vi "PullZeros.vi"(4 "input":dbl[](array[numeric]) format="%.2f") -> (0 "output":dbl[](array[numeric]) format="%.2f", 1 "non zero points":i32, 2 "pre-zeros":i32)   [LabVIEW 2022 SP3]
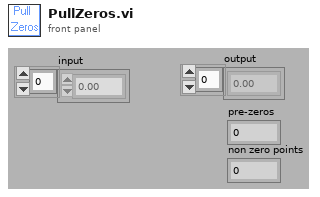
[diagram p1: front panel]
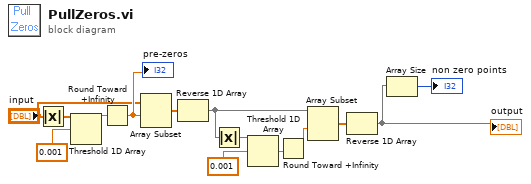
[diagram p0: block diagram]
diagram:
  n1 = Absolute Value(x="input") -> (abs(x)=w3:dbl[])
  n2 = Threshold 1D Array(2:0.001, 3:w3) -> (0:w10:dbl)  [unwired: 1 out]
  n3 = Round Toward +Infinity(x=w10) -> (ceil(x): smallest int >= x=w14:dbl)
  "pre-zeros" <- w14
  n4 = Array Subset(array="input", index=w14) -> (w4:dbl[])  [unwired: 1 in]
  n5 = Reverse 1D Array(array=w4) -> (reversed array=w7:dbl[])
  n6 = Absolute Value(x=w7) -> (abs(x)=w6:dbl[])
  n7 = Threshold 1D Array(2:0.001, 3:w6) -> (0:w9:dbl)  [unwired: 1 out]
  n8 = Round Toward +Infinity(x=w9) -> (ceil(x): smallest int >= x=w12:dbl)
  n9 = Array Subset(array=w7, index=w12) -> (w8:dbl[])  [unwired: 1 in]
  n10 = Reverse 1D Array(array=w8) -> (reversed array=w1:dbl[])
  "output" <- w1
  n11 = Array Size(array=w1) -> (size(s)=→"non zero points":i32)
